vi "Main (1553).vi"() -> ()   [LabVIEW 2020]
doc: "Use this template to build a simple state machine design pattern. Each state executes code and determines which state to transition to."
uses:
  Controls/Encoding.ctl
  Controls/Database_Array.ctl
  <userlib>/_OpenG.lib/array/array.llb/Remove Duplicates from 1D Array (I32)__ogtk.vi
  <userlib>/_OpenG.lib/array/array.llb/Sort 1D Array (I32)__ogtk.vi
  <userlib>/_OpenG.lib/array/array.llb/Index 1D Array Elements (Variant)__ogtk.vi
  <userlib>/_OpenG.lib/array/array.llb/Search 1D Array (I32)__ogtk.vi
  <vilib>/Utility/error.llb/DialogType.ctl
  Libraries/Ballard_Parameter_ni/Ballard_429_Parameter_ni.lvlib
  1553/_controls/1553_State.ctl
  1553/_controls/1553_formatting.ctl
  1553/_controls/1553_Data.ctl
  1553/_controls/1553_Frames.ctl
  1553/_controls/1553_Parameters.ctl
  1553/_controls/1553_Parameters_key.ctl
  1553/_controls/1553_messages.ctl
  1553/_controls/aim1553_cluster.ctl
  Libraries/Aim_1553_Parameter_ni/AIM_1553_Parameter_ni.lvlib
panel:
  in  "formatting":T1
  in  "Configure SelfTestBus?":bool
  out "Progress":string
  in  "Stop Button":bool
  in  "Generate XMLs":bool
  in  "Database Filepath (xlsx)":path
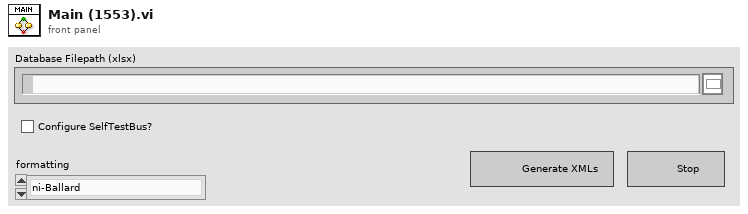
[diagram p1: front panel]
types:
  T1 = typedef "1553_formatting.ctl" = enum16{"ni-Ballard", "ni-AIM"}
  T2 = typedef "DialogType.ctl" = u16
  T3 = typedef "1553_Data.ctl" = cluster{"Cores to Process Array":i32[], "All Parameters Array":T4[], "Filtered Parameter Array":T4[], "Core Number":i32, "Database Filepath (xlsx)":path, "Selected Self Test Channels":i32[], "formatting":T1, "aim1553_cluster":T6}
  T4 = typedef "Database_Array.ctl" = cluster{"Core Number":i32, "Channel Number":i32, "Channel Name":string, "Channel Speed":i32, "Label Decimal":i32, "Label Name":string, "Min Rate (mS)":i32, "Max Rate (mS)":i32, "SDI":i32, "SSM":i32, "Create SDI":bool, "Create SSM":bool, "Create Parity":bool, "Parameter Name":string, "Start Bit":i32, "Number of Bits":i32, "Scale":string, "Offset":string, "Signed":bool, "Unit":string, "Encoding":T5, "Default Value":string}
  T5 = typedef "Encoding.ctl" = enum16{"BCD", "BNR", "Discrete"}
  T6 = typedef "aim1553_cluster.ctl" = cluster{"messages":map{string, T7}, "parameters":map{T8, T9[]}, "frames":map{string, T10}}
  T7 = typedef "1553_messages.ctl" = cluster{"messageType":string, "TA1":i32, "SA1":i32, "words":i32, "TA2":i32, "SA2":i32, "MC":i32, "direction":string}
  T8 = typedef "1553_Parameters_key.ctl" = cluster{"TA":i32, "SA":i32}
  T9 = typedef "1553_Parameters.ctl" = cluster{"name":string, "encoding":string, "signed":bool, "startBit":i32, "numberOfBits":i32, "scale":dbl, "offset":dbl, "unit":string, "defaultValue":dbl}
  T10 = typedef "1553_Frames.ctl" = cluster{"MinorFrameName":string, "MajorFrameName":string, "FramePeriodUs":i32}
  T11 = typedef "1553_State.ctl" = enum16{"Initialize", "Wait for Event", "Read Database File", "Get Core Data", "Write HW XML File", "Write Parameter XML File", "Exit"}
  T12 = enum8{"Enabled", "Disabled", "Disabled and Grayed Out"}
  T13 = enum32{"invalid app kind", "Development System", "Run Time System", "Student Edition", "Embedded LabVIEW", "Evaluation", "Custom"}
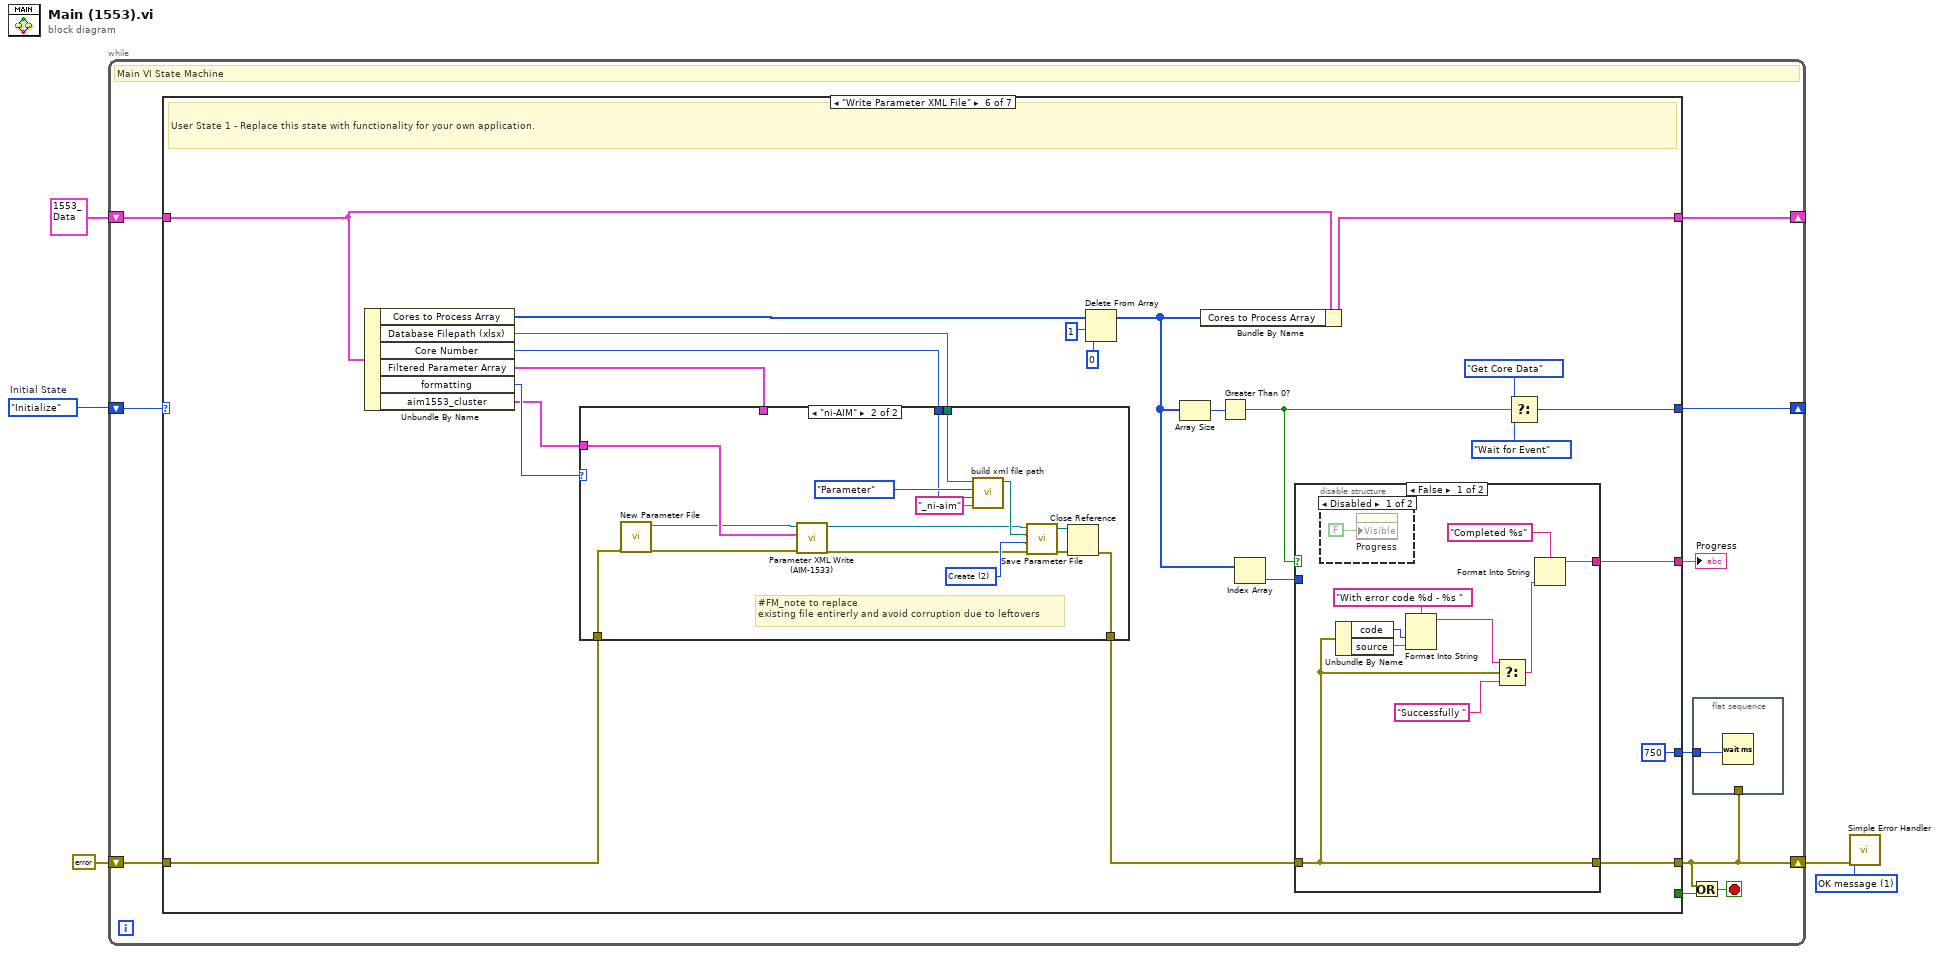
[diagram p0: block diagram]
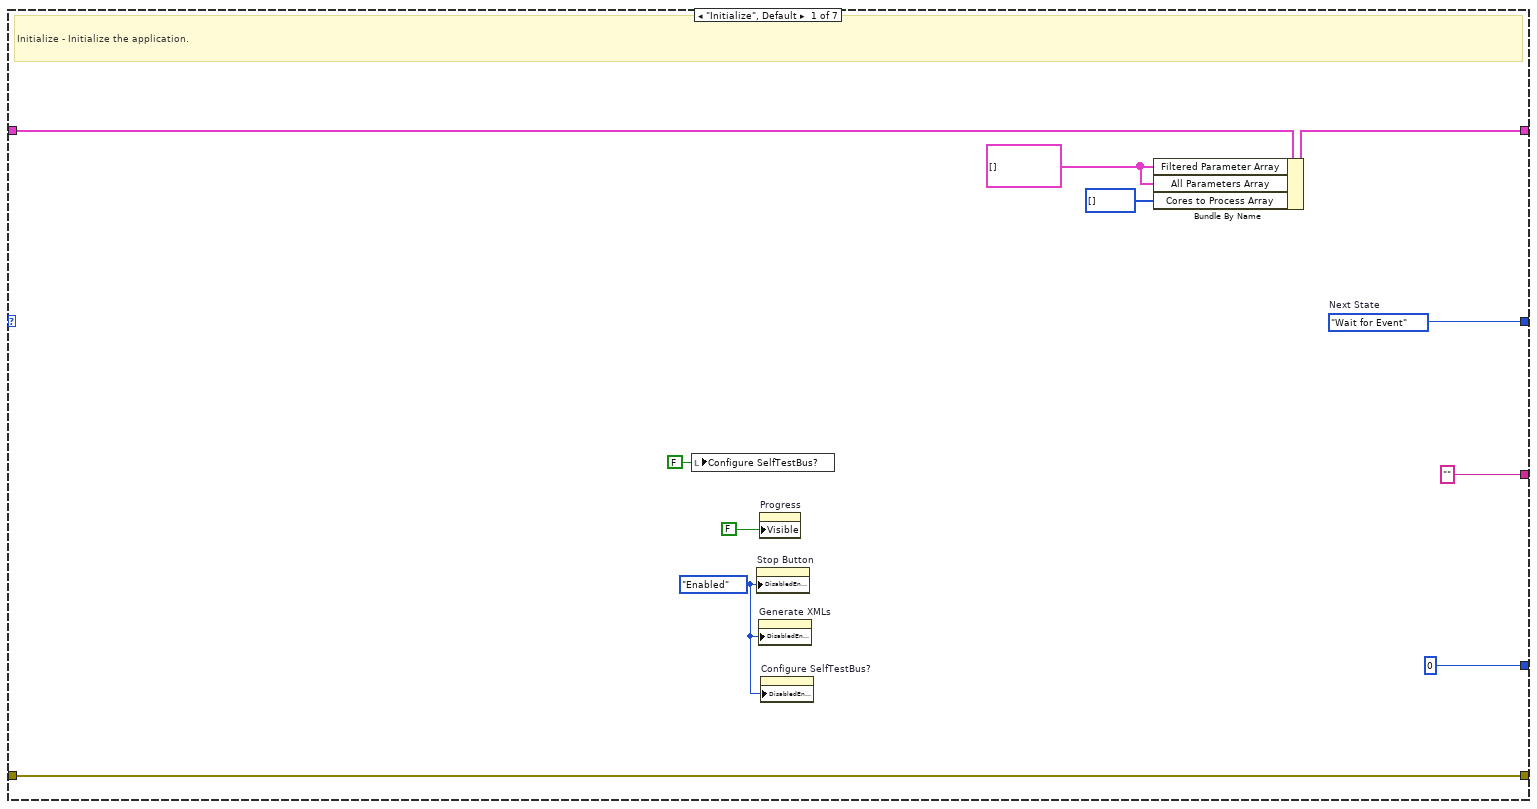
[diagram p2: hidden frame]
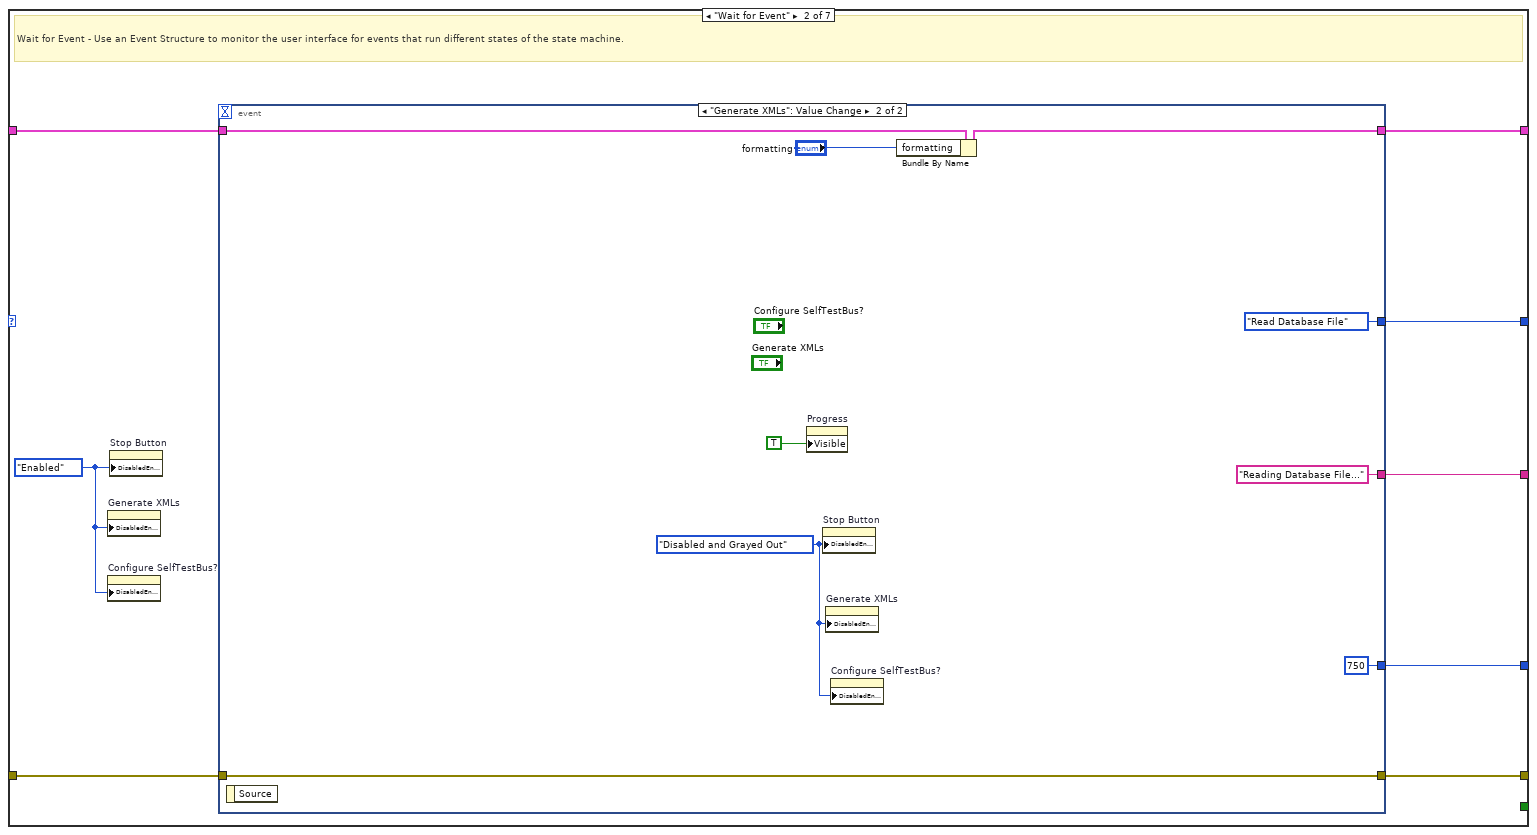
[diagram p3: hidden frame]
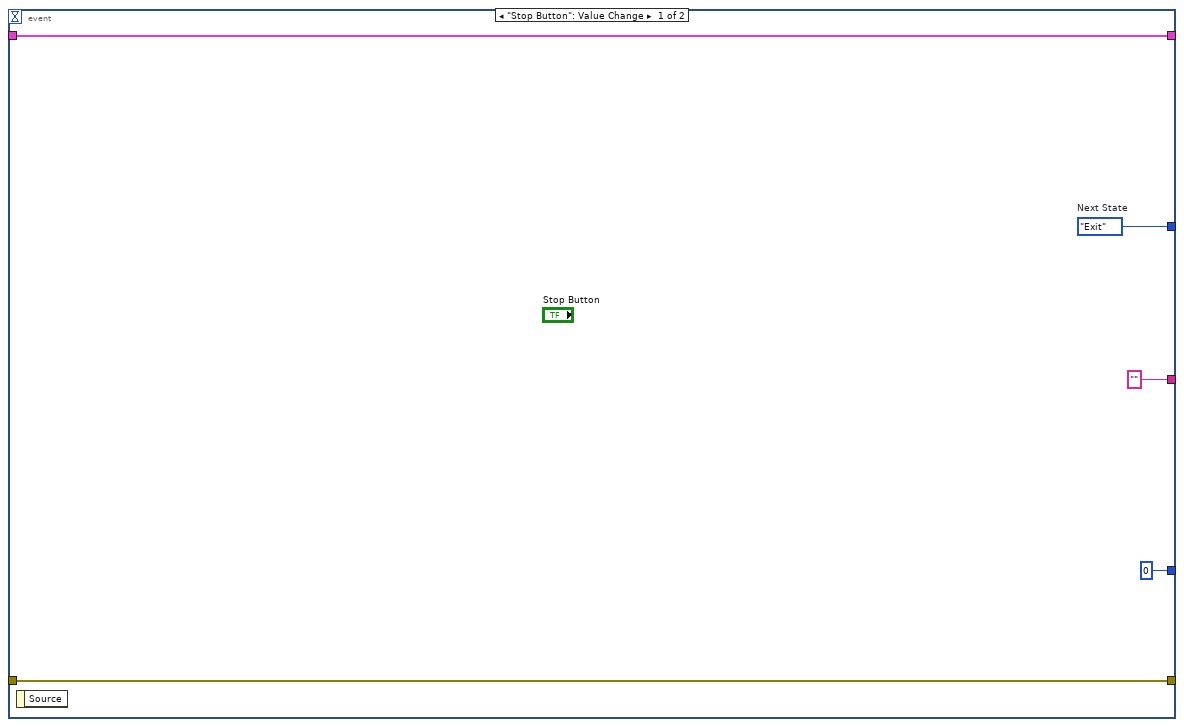
[diagram p4: hidden frame]
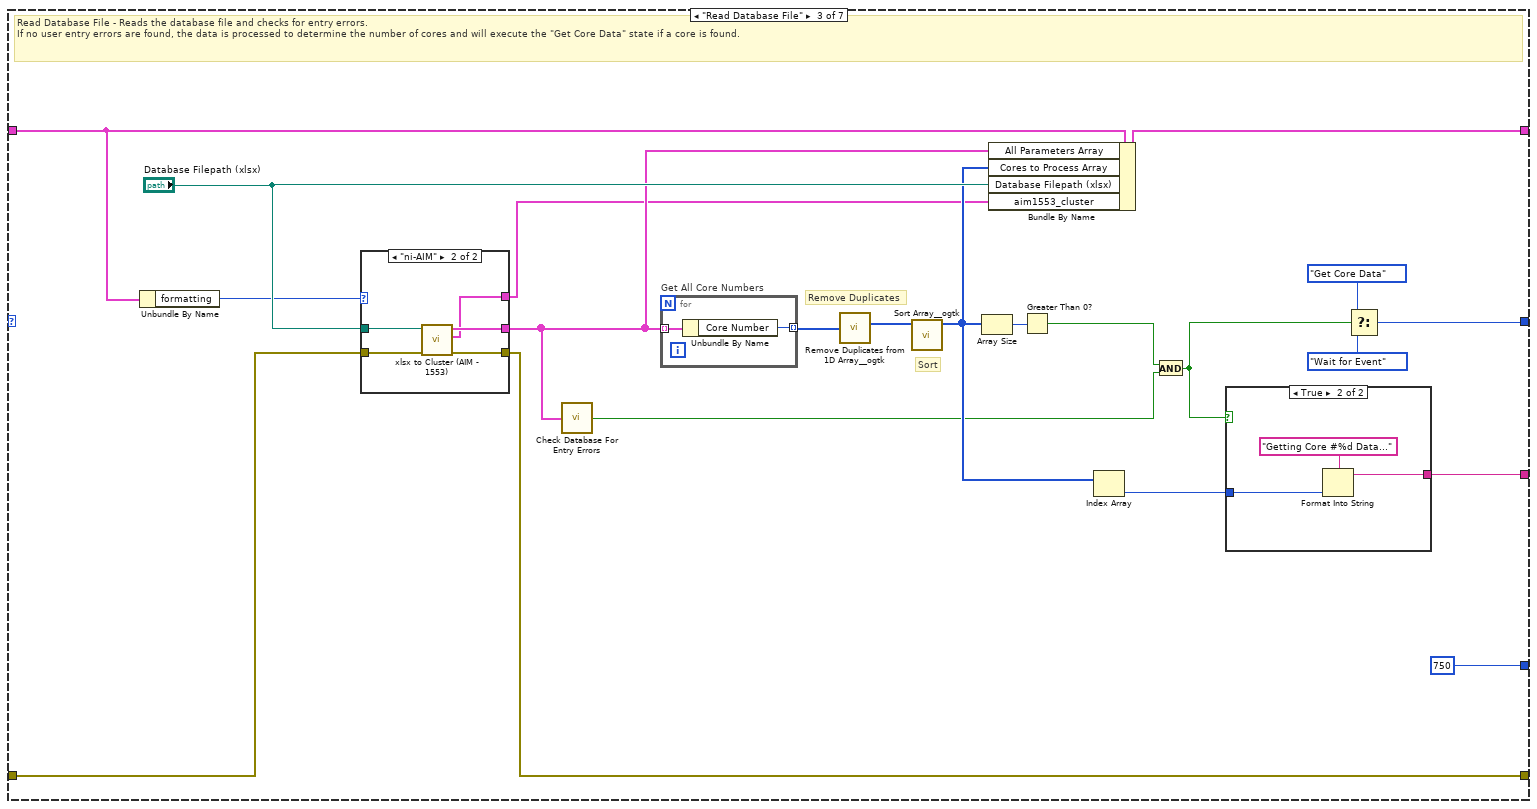
[diagram p5: hidden frame]
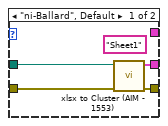
[diagram p6: hidden frame]
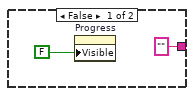
[diagram p7: hidden frame]
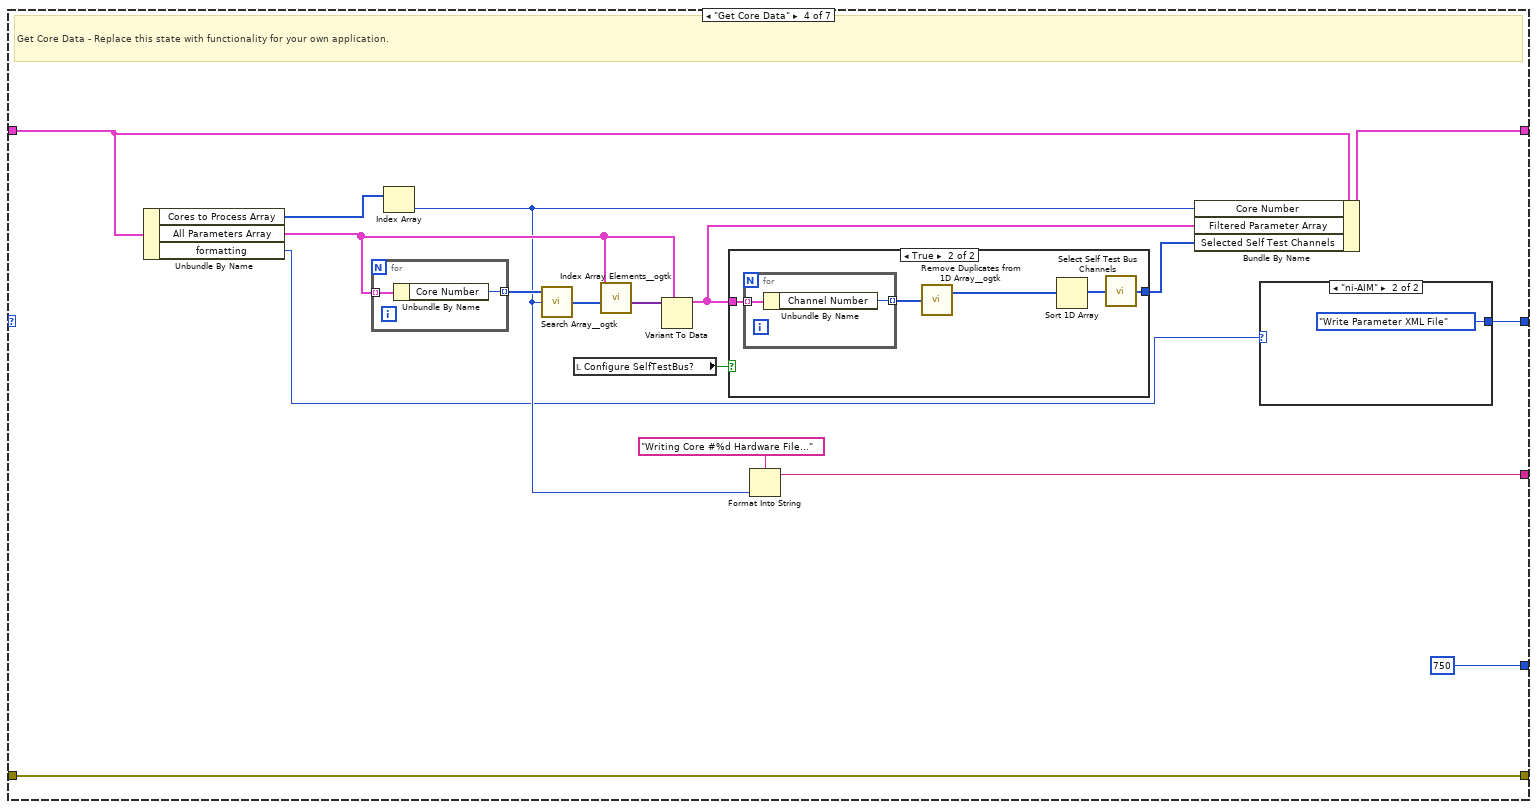
[diagram p8: hidden frame]
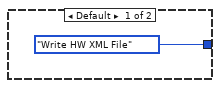
[diagram p9: hidden frame]
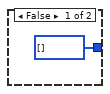
[diagram p10: hidden frame]
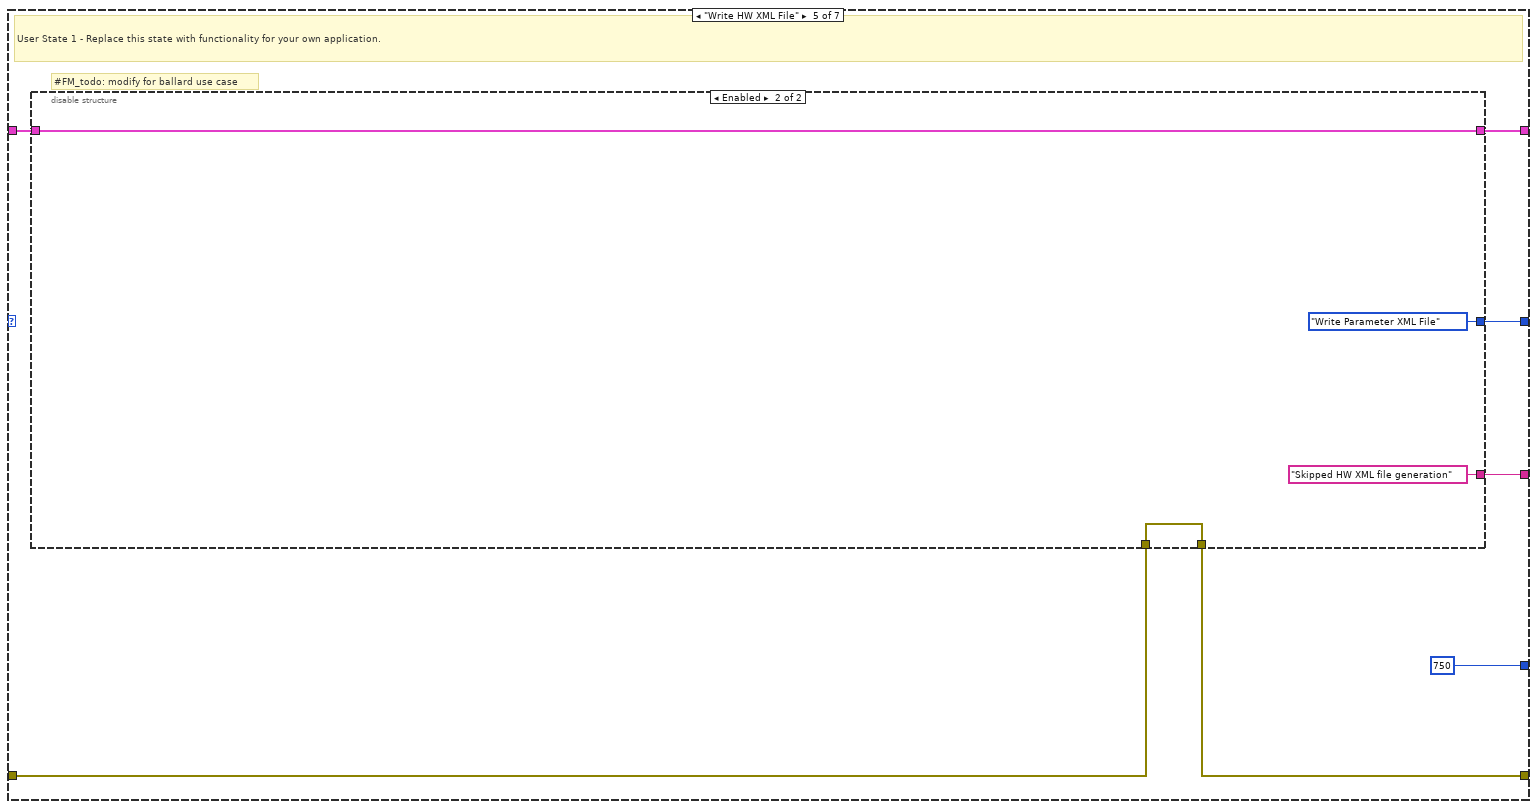
[diagram p11: hidden frame]
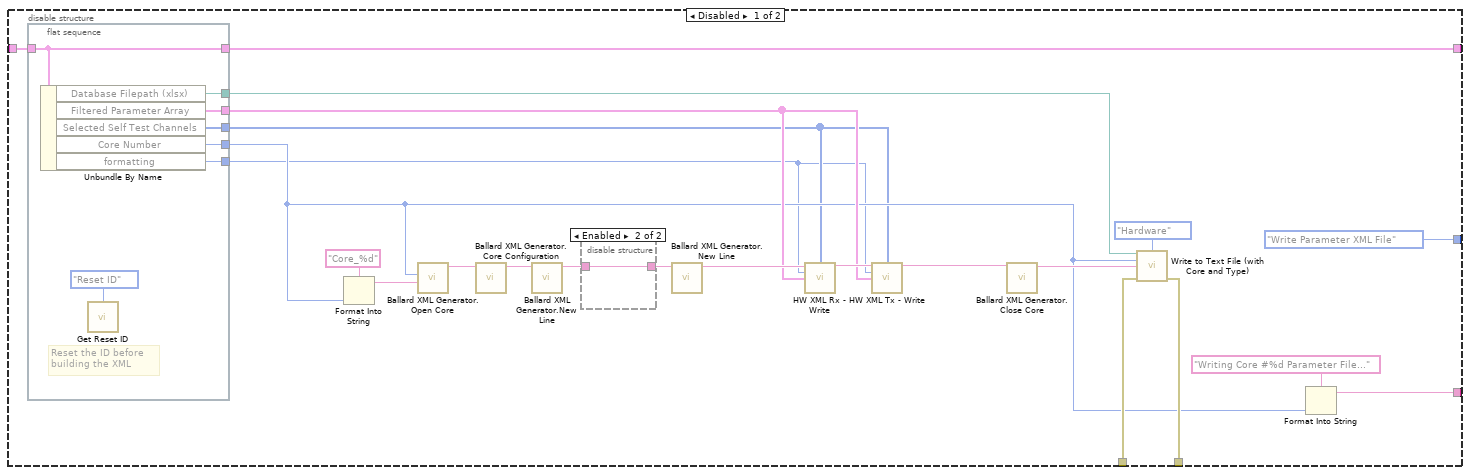
[diagram p12: hidden frame]
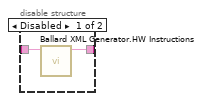
[diagram p13: hidden frame]
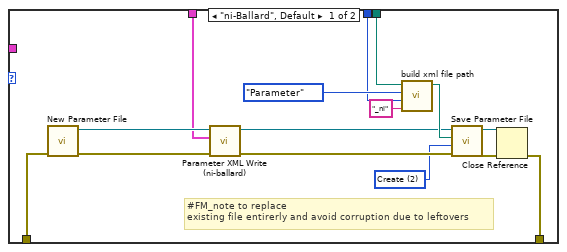
[diagram p14: hidden frame]
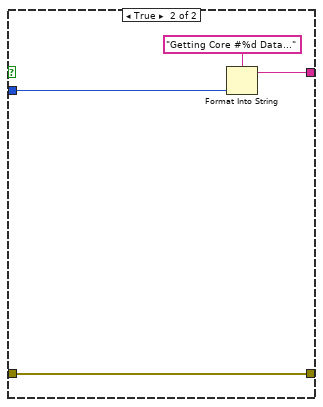
[diagram p16: hidden frame]
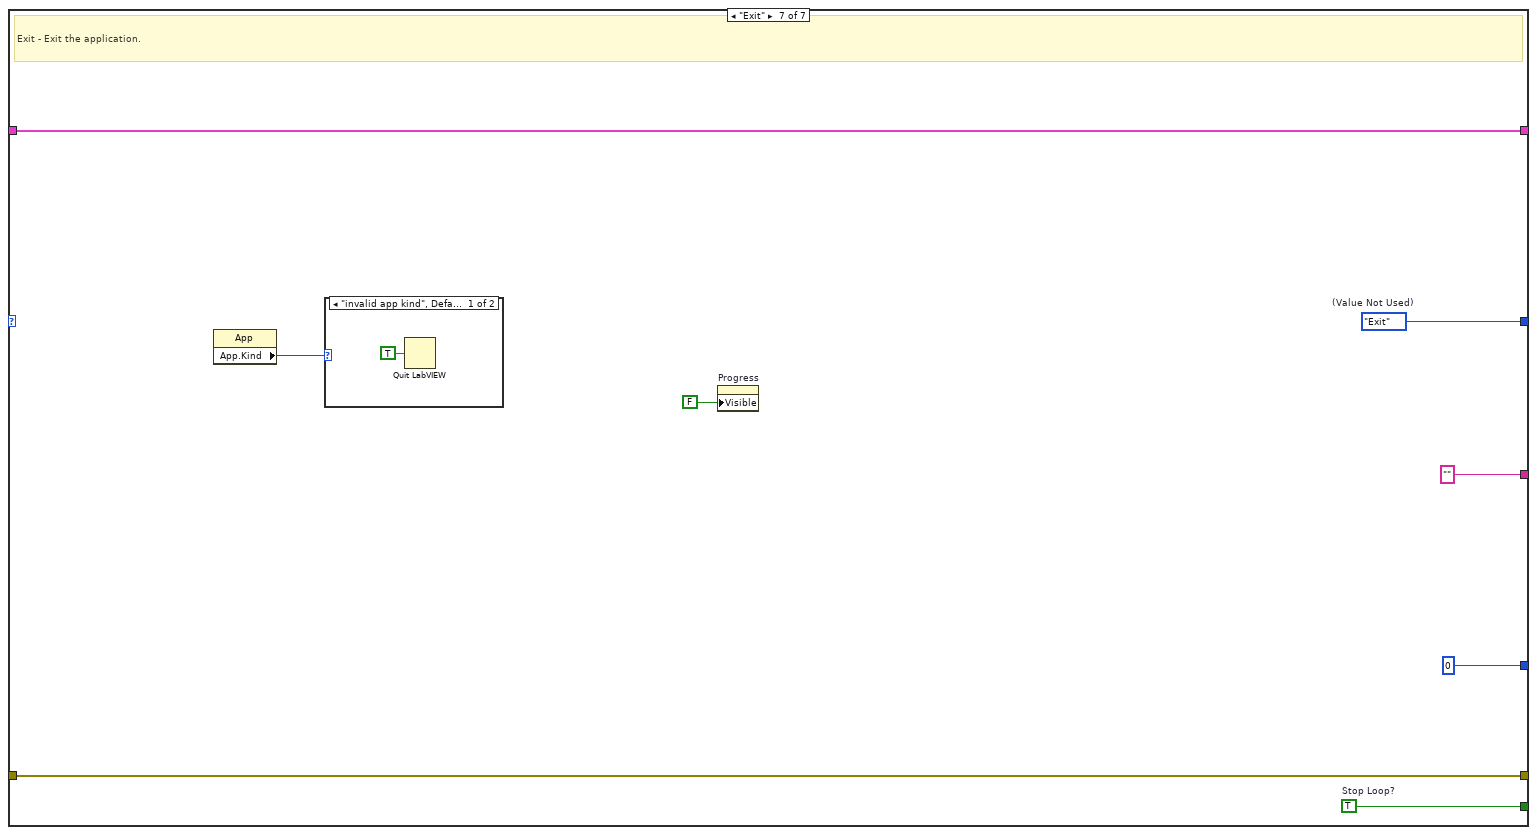
[diagram p17: hidden frame]
diagram:
  w1 = T2 1 items=["no dialog", "OK message", "continue or stop message", "OK message + warnings", "continue/stop + warnings"] ("type of dialog (OK msg:1)")
  w5 = 1553_State."Initialize"  # Initial State
  n1 = while {
    shift-right: [w14] -> _
    shift-left: w5 -> [w15]
    shift-right: [w12] -> _
    shift-left: T3 {"Cores to Process Array"=[], "All Parameters Array"=[], "Filtered Parameter Array"=[], "Core Number"=0, "Database Filepath (xlsx)"=path "C:/Users/jkreienh/Desktop/Preliminary Ballard Database Template.xlsx", "Selected Self Test Channels"=[], "formatting"=enum."ni-Ballard", "aim1553_cluster"={"messages"={}, "parameters"={}, "frames"={}}} ("Data") -> [w13]
    shift-right: [w7] -> w2
    shift-left: errorcluster {"status"=FALSE, "code"=0, "source"=""} ("error constant") -> [w11]
    stop <- w9 stop-if-true
    # "Main VI State Machine"
    n2 = case shown="\"Write Parameter XML File\"" w15 {
      tunnel: [w27 w35 w63 w97 w122 w177 w233] -> w14
      tunnel: [_ _ _ _ _ _ w231] -> w10
      tunnel: w13 -> [w25 w34 w52 w101 w119 w174 w232]
      tunnel: [w24 w33 w67 w91 w118 w173 w232] -> w12
      tunnel: w11 -> [w26 w32 w60 w96 w121 w181 w230]
      tunnel: [w26 w31 w70 w96 w120 w162 w230] -> w7
      tunnel: ["" w30 w59 w93 w117 w169 ""] -> w8
      tunnel: [u32 0 ("milliseconds to wait") w29 u32 750 ("milliseconds to wait") u32 750 ("milliseconds to wait") u32 750 ("milliseconds to wait") u32 750 ("milliseconds to wait") u32 0 ("milliseconds to wait")] -> w6
      frame "Initialize", Default {
        w18 = T12."Enabled" ("Disabled")
        w22 = T4[] [] ("Parameter Array")
        w27 = 1553_State."Wait for Event"  # Next State
        # "Initialize - Initialize the application."
        n3 = local write "Configure SelfTestBus?"(FALSE ("Configure SelfTestBus?")) -> ()
        n4 = property on="Stop Button" class="Bool"("DisabledEnum"=w18) -> ()  [unwired: 2 in, 2 out]
        n5 = property on="Generate XMLs" class="Bool"("DisabledEnum"=w18) -> ()  [unwired: 2 in, 2 out]
        n6 = property on="Progress" class="Str"("Visible"=FALSE) -> ()  [unwired: 2 in, 2 out]
        n7 = property on="Configure SelfTestBus?" class="Bool (strict)"("DisabledEnum"=w18) -> ()  [unwired: 2 in, 2 out]
        n8 = Bundle By Name(cluster=w25, "Filtered Parameter Array"=w22, "All Parameters Array"=w22, "Cores to Process Array"=i32[] [] ("Core Array")) -> (w24:T3)
      }
      frame "Wait for Event" {
        w28 = T12."Enabled" ("Disabled")
        # "Wait for Event - Use an Event Structure to monitor the user interface for events that run different states of the state machine."
        n9 = property on="Generate XMLs" class="Bool"("DisabledEnum"=w28) -> ()  [unwired: 2 in, 2 out]
        n10 = property on="Configure SelfTestBus?" class="Bool (strict)"("DisabledEnum"=w28) -> ()  [unwired: 2 in, 2 out]
        n11 = property on="Stop Button" class="Bool"("DisabledEnum"=w28) -> ()  [unwired: 2 in, 2 out]
        n12 = event shown="[1] \"Generate XMLs\": Value Change" {
          selector: _ -> [_ _]
          dyn-events: _ -> [_ _]
          timeout: _ -> [_ _]
          tunnel: [w40 1553_State."Read Database File" ("Next State")] -> w35
          tunnel: w34 -> [w39 w49]
          tunnel: [w39 w42] -> w33
          tunnel: w32 -> [w38 w48]
          tunnel: [w38 w48] -> w31
          tunnel: ["" "Reading Database File..."] -> w30
          tunnel: [u32 0 ("milliseconds to wait") u32 750 ("milliseconds to wait")] -> w29
          event "Stop Button": Value Change {
            w40 = 1553_State."Exit"  # Next State
            n13 = event-data() -> ()  [unwired: 1 in, 1 out]
          }
          event "Generate XMLs": Value Change {
            w43 = T12."Disabled and Grayed Out" ("Disabled")
            n14 = event-data() -> ()  [unwired: 1 in, 1 out]
            n15 = property on="Progress" class="Str"("Visible"=TRUE) -> ()  [unwired: 2 in, 2 out]
            n16 = property on="Stop Button" class="Bool"("DisabledEnum"=w43) -> ()  [unwired: 2 in, 2 out]
            n17 = property on="Generate XMLs" class="Bool"("DisabledEnum"=w43) -> ()  [unwired: 2 in, 2 out]
            n18 = property on="Configure SelfTestBus?" class="Bool (strict)"("DisabledEnum"=w43) -> ()  [unwired: 2 in, 2 out]
            n19 = Bundle By Name(cluster=w49, "formatting"="formatting") -> (w42:T3)
          }
        }
      }
      frame "Read Database File" {
        # "Sort"
        # "Remove Duplicates"
        # "Read Database File - Reads the database file and checks for entry errors. \nIf no user entry errors are found, the data is processed to determine the number of cores and will execute the \"Get Core Data\" state if a core is found."
        n20 = Unbundle By Name(w52) -> ("formatting"=w51:T1)
        n21 = case shown="\"ni-AIM\"" w51 {
          tunnel: [w74 w77] -> w70
          tunnel: "Database Filepath (xlsx)" -> [w73 w79]
          tunnel: [w72 w76] -> w61
          tunnel: w60 -> [w71 w78]
          tunnel: [_ w75] -> w50
          frame "ni-Ballard", Default {
            (unwired) "Sheet1" ("Excel._SheetName")
            n22 = call "xlsx to Cluster (AIM - 1553).vi"("Error (in)"=w71, "file path (dialog if empty)"=w73) -> ("Error (out)"=w74:errorcluster, "Parameter Array"=w72:T4[])  [unwired: 7 in, 1 out]
          }
          frame "ni-AIM" {
            n23 = call "xlsx to Cluster (AIM - 1553).vi"("Error (in)"=w78, "file path (dialog if empty)"=w79) -> ("Error (out)"=w77:errorcluster, "aim1553_cluster"=w75:T6, "Parameter Array"=w76:T4[])  [unwired: 7 in]
          }
        }
        n24 = call "Check Database For Entry Errors.vi"("All Parameters Array"=w61) -> ("Database OK?"=w54:bool)  [unwired: 14 in]
        n25 = for "Get All Core Numbers" {
          tunnel: w61 -> [w86] mode=indexing
          tunnel: [w85] -> w69 mode=indexing
          n26 = Unbundle By Name(w86) -> ("Core Number"=w85:i32)
        }
        n27 = call-poly <userlib>:"Remove Duplicates from 1D Array__ogtk.vi"("Input Array"=w69) -> ("Output Array"=w68:i32[])  [unwired: 1 out]
        n28 = call-poly <userlib>:"Sort Array__ogtk.vi"("Array in"=w68) -> ("Sorted Array out"=w58:i32[])  [unwired: 9 in, 1 out]
        n29 = Array Size(array=w58) -> (size(s)=w66:i32)
        n30 = Bundle By Name(cluster=w52, "All Parameters Array"=w61, "Cores to Process Array"=w58, "Database Filepath (xlsx)"="Database Filepath (xlsx)", "aim1553_cluster"=w50) -> (w67:T3)
        n31 = Greater Than 0?(x=w66) -> (x > 0?=w55:bool)
        n32 = Index Array(array=w58) -> (element=w57:i32)  [unwired: 1 in]
        n33 = And(x=w55, y=w54) -> (x .and. y?=w53:bool)
        n34 = case shown="True" w53 {
          tunnel: ["" ("f") w83] -> w59
          tunnel: w57 -> [_ w84]
          frame False {
            n35 = property on="Progress" class="Str"("Visible"=FALSE) -> ()  [unwired: 2 in, 2 out]
          }
          frame True {
            n36 = Format Into String(format string="Getting Core #%d Data..." ("String"), w84) -> (resulting string=w83:string)  [unwired: 2 in, 1 out]
          }
        }
        n37 = Select(t=1553_State."Get Core Data", s=w53, f=1553_State."Wait for Event") -> (s? t:f=w63:T11)
      }
      frame "Get Core Data" {
        # "Get Core Data - Replace this state with functionality for your own application."
        n38 = Unbundle By Name(w101) -> ("Cores to Process Array"=w98:i32[], "All Parameters Array"=w100:T4[], "formatting"=w87:T1)
        n39 = for {
          tunnel: w100 -> [w115] mode=indexing
          tunnel: [w114] -> w103 mode=indexing
          n40 = Unbundle By Name(w115) -> ("Core Number"=w114:i32)
        }
        n41 = Index Array(array=w98) -> (element=w94:i32)  [unwired: 1 in]
        n42 = call-poly <userlib>:"Search Array__ogtk.vi"("Array"=w103, "Element Data"=w94) -> ("Indices of Elements"=w102:i32[])  [unwired: 7 in]
        n43 = local read "Configure SelfTestBus?"() -> (w88:bool)
        n44 = call-poly <userlib>:"Index Array Elements__ogtk.vi"("indices"=w102, "array"=w100) -> ("elements"=w99:variant[])  [unwired: 9 in]
        n45 = Variant To Data(type=w100, Variant=w99) -> (data=w90:T4[])  [unwired: 1 in, 1 out]
        n46 = case shown="True" w88 {
          tunnel: w90 -> [_ w110]
          tunnel: [i32[] [] ("Selected Channels") w107] -> w89
          frame False {
          }
          frame True {
            n47 = for {
              tunnel: [w113] -> w109 mode=indexing
              tunnel: w110 -> [w112] mode=indexing
              n48 = Unbundle By Name(w112) -> ("Channel Number"=w113:i32)
            }
            n49 = call-poly <userlib>:"Remove Duplicates from 1D Array__ogtk.vi"("Input Array"=w109) -> ("Output Array"=w111:i32[])  [unwired: 1 out]
            n50 = Sort 1D Array(array=w111) -> (sorted array=w108:i32[])
            n51 = call "Select Self Test Bus Channels.vi"("Channels"=w108) -> ("Selected Channels"=w107:i32[])  [unwired: 14 in]
          }
        }
        n52 = Format Into String(format string="Writing Core #%d Hardware File..." ("String"), w94) -> (resulting string=w93:string)  [unwired: 2 in, 1 out]
        n53 = Bundle By Name(cluster=w101, "Core Number"=w94, "Filtered Parameter Array"=w90, "Selected Self Test Channels"=w89) -> (w91:T3)
        n54 = case shown="\"ni-AIM\"" w87 {
          tunnel: [1553_State."Write HW XML File" 1553_State."Write Parameter XML File"] -> w97
          frame Default {
          }
          frame "ni-AIM" {
          }
        }
      }
      frame "Write HW XML File" {
        # "#FM_todo: modify for ballard use case"
        # "User State 1 - Replace this state with functionality for your own application."
        n55 = disable-structure shown="Enabled" {
          disable-tunnel: [1553_State."Write Parameter XML File" ("Next State") 1553_State."Write Parameter XML File" ("Next State")] -> w122
          disable-tunnel: w121 -> [w133 w157]
          disable-tunnel: [w132 w157] -> w120
          disable-tunnel: w119 -> [w130 w158]
          disable-tunnel: [w129 w158] -> w118
          disable-tunnel: [w126 "Skipped HW XML file generation"] -> w117
          frame Disabled {
            n56 = flat-sequence {
              tunnel: [w152] -> w135
              tunnel: w130 -> [w150]
              tunnel: [w150] -> w129
              tunnel: [w149] -> w128
              tunnel: [w148] -> w125
              tunnel: [w147] -> w124
              tunnel: [w146] -> w123
              frame #0 {
                # "Reset the ID before building the XML"
                n57 = Unbundle By Name(w150) -> ("Database Filepath (xlsx)"=w149:path, "Filtered Parameter Array"=w152:T4[], "Selected Self Test Channels"=w147:i32[], "Core Number"=w148:i32, "formatting"=w146:T1)
                n58 = call "Get Reset ID.vi"("Function"=enum16{"Get ID", "Reset ID"}."Reset ID") -> ()  [unwired: 14 in, 1 out]
              }
            }
            n59 = Format Into String(format string="Core_%d", w125) -> (resulting string=w136:string)  [unwired: 2 in, 1 out]
            n60 = call "Ballard XML Generator.Open Core.vi"("name"=w136, "id"=w125) -> ("string out"=w138:string)  [unwired: 9 in]
            n61 = call "Ballard XML Generator.Core Configuration.vi"("string in"=w138) -> ("string out"=w139:string)  [unwired: 10 in]
            n62 = call "Ballard XML Generator.New Line.vi"("string in"=w139) -> ("string out"=w140:string)  [unwired: 10 in]
            n63 = disable-structure shown="Enabled" {
              disable-tunnel: w140 -> [w154 w155]
              disable-tunnel: [w153 w155] -> w141
              frame Disabled {
                n64 = call "Ballard XML Generator.HW Instructions.vi"("string in"=w154) -> ("string out"=w153:string)  [unwired: 10 in]
              }
              frame Enabled {
              }
            }
            n65 = call "Ballard XML Generator.New Line.vi"("string in"=w141) -> ("string out"=w142:string)  [unwired: 10 in]
            n66 = call "HW XML Rx - Write.vi"("String (in)"=w142, "Selected Channels"=w124, "formatting (NIVeriStandAdd-Ons)"=w123, "Parameter Array"=w135) -> ("String (out)"=w143:string)  [unwired: 11 in]
            n67 = call "HW XML Tx - Write.vi"("String (in)"=w143, "Selected Channels"=w124, "formatting (NIVeriStandAdd-Ons)"=w123, "Parameter Array"=w135) -> ("String (out)"=w144:string)  [unwired: 11 in]
            n68 = call "Ballard XML Generator.Close Core.vi"("string in"=w144) -> ("string out"=w131:string)  [unwired: 10 in]
            n69 = call "Write to Text File (with Core and Type).vi"("Database Filepath (xlsx)"=w128, "Filetype"=enum16{"Hardware", "Parameter"}."Hardware", "Core"=w125, "Text"=w131, "Error (in)"=w133) -> ("Error (out)"=w132:errorcluster)  [unwired: 10 in]
            n70 = Format Into String(format string="Writing Core #%d Parameter File..." ("String"), w125) -> (resulting string=w126:string)  [unwired: 2 in, 1 out]
          }
          frame Enabled {
          }
        }
      }
      frame "Write Parameter XML File" {
        # "User State 1 - Replace this state with functionality for your own application."
        n71 = Unbundle By Name(w174) -> ("Cores to Process Array"=w175:i32[], "Database Filepath (xlsx)"=w171:path, "Core Number"=w168:i32, "Filtered Parameter Array"=w172:T4[], "formatting"=w161:T1, "aim1553_cluster"=w160:T6)
        n72 = case shown="\"ni-AIM\"" w161 {
          tunnel: w181 -> [w196 w205]
          tunnel: [w195 w211] -> w163
          tunnel: w172 -> [w186 _]
          tunnel: w171 -> [w191 w209]
          tunnel: w168 -> [w190 w208]
          tunnel: w160 -> [_ w206]
          frame "ni-Ballard", Default {
            w182 = 2 items=["CreateNew"=1, "Create"=2, "Open"=3, "OpenOrCreate"=4, "Truncate"=5, "Append"=6] ("mode (Create)")
            # "#FM_note to replace \nexisting file entirerly and avoid corruption due to leftovers"
            n73 = call "New Parameter File.vi"("error in"=w196) -> ("error out"=w187:errorcluster, "new parameter file"=w188:refnum<k24>)  [unwired: 9 in]
            n74 = call "Parameter XML Write (ni-ballard).vi"("error in"=w187, "Parameter Array"=w186, "parameter file in"=w188) -> ("error out"=w184:errorcluster, "parameter file out"=w185:refnum<k24>)  [unwired: 7 in]
            n75 = call "build xml file path.vi"("additional string(\"\")"="_ni" ("additional string(\"\")"), "Core"=w190, "Filetype"=enum16{"Hardware", "Parameter"}."Parameter", "Database Filepath in"=w191) -> ("xml path out"=w189:path)  [unwired: 7 in]
            n76 = call "Save Parameter File.vi"("error in"=w184, "mode (Create)"=w182, "XML path"=w189, "parameter file in"=w185) -> ("error out"=w194:errorcluster, "parameter file out"=w193:refnum<k24>)  [unwired: 5 in, 1 out]
            n77 = Close Reference(reference=w193, error in (no error)=w194) -> (error out=w195:errorcluster)
          }
          frame "ni-AIM" {
            w202 = 2 items=["CreateNew"=1, "Create"=2, "Open"=3, "OpenOrCreate"=4, "Truncate"=5, "Append"=6] ("mode (Create)")
            # "#FM_note to replace \nexisting file entirerly and avoid corruption due to leftovers"
            n78 = call "New Parameter File.vi"("error in"=w205) -> ("error out"=w198:errorcluster, "new parameter file"=w197:refnum<k24>)  [unwired: 9 in]
            n79 = call "Parameter XML Write (AIM-1533).vi"("error in"=w198, "aim1553_cluster"=w206, "parameter file in"=w197) -> ("error out"=w200:errorcluster, "parameter file out"=w199:refnum<k24>)  [unwired: 7 in]
            n80 = call "build xml file path.vi"("additional string(\"\")"="_ni-aim" ("additional string(\"\")"), "Core"=w208, "Filetype"=enum16{"Hardware", "Parameter"}."Parameter", "Database Filepath in"=w209) -> ("xml path out"=w201:path)  [unwired: 7 in]
            n81 = call "Save Parameter File.vi"("error in"=w200, "mode (Create)"=w202, "XML path"=w201, "parameter file in"=w199) -> ("error out"=w204:errorcluster, "parameter file out"=w203:refnum<k24>)  [unwired: 5 in, 1 out]
            n82 = Close Reference(reference=w203, error in (no error)=w204) -> (error out=w211:errorcluster)
          }
        }
        n83 = Delete From Array(array=w175, length=1, index=0) -> (array with subset deleted=w166:i32[])  [unwired: 1 out]
        n84 = Array Size(array=w166) -> (size(s)=w180:i32)
        n85 = Bundle By Name(cluster=w174, "Cores to Process Array"=w166) -> (w173:T3)
        n86 = Greater Than 0?(x=w180) -> (x > 0?=w167:bool)
        n87 = Index Array(array=w166) -> (element=w165:i32)  [unwired: 1 in]
        n88 = case shown="False" w167 {
          tunnel: [w219 w224] -> w169
          tunnel: w165 -> [_ w223]
          tunnel: w163 -> [w212 w222]
          tunnel: [w212 w222] -> w162
          frame False {
            n89 = disable-structure shown="Disabled" {
              frame Disabled {
                n90 = property on="Progress" class="Str"("Visible"=FALSE) -> ()  [unwired: 2 in, 2 out]
              }
              frame Enabled {
              }
            }
            n91 = Unbundle By Name(w212) -> ("code"=w217:i32, "source"=w216:string)
            n92 = Format Into String(format string="With error code %d - %s ", w217, w216) -> (resulting string=w214:string)  [unwired: 2 in, 1 out]
            n93 = Select(t=w214, s=w212, f="Successfully ") -> (s? t:f=w215:string)
            n94 = Format Into String(format string="Completed %s", w215) -> (resulting string=w219:string)  [unwired: 2 in, 1 out]
          }
          frame True {
            n95 = Format Into String(format string="Getting Core #%d Data..." ("String"), w223) -> (resulting string=w224:string)  [unwired: 2 in, 1 out]
          }
        }
        n96 = Select(t=1553_State."Get Core Data" ("Next State"), s=w167, f=1553_State."Wait for Event" ("Next State")) -> (s? t:f=w177:T11)
      }
      frame "Exit" {
        w231 = TRUE  # Stop Loop?
        w233 = 1553_State."Exit"  # (Value Not Used)
        # "Exit - Exit the application."
        n97 = property class="App"() -> ("App.Kind"=w226:T13)  [unwired: 2 in, 2 out]
        n98 = case shown="\"invalid app kind\", Default" w226 {
          frame "invalid app kind", Default {
            n99 = Quit LabVIEW(quit? (T)=TRUE) -> ()
          }
          frame "Development System" {
          }
        }
        n100 = property on="Progress" class="Str"("Visible"=FALSE) -> ()  [unwired: 2 in, 2 out]
      }
    }
    "Progress" <- w8
    n101 = Or(x=w7, y=w10) -> (x .or. y?=w9:bool)
    n102 = flat-sequence {
      tunnel: w7 -> [_]
      tunnel: w6 -> [w16]
      frame #0 {
        n103 = Wait (ms)(milliseconds to wait=w16) -> ()  [unwired: 1 out]
      }
    }
  }
  n104 = call <vilib>:"Simple Error Handler.vi"("type of dialog (OK msg:1)"=w1, "error in (no error)"=w2) -> ()  [unwired: 3 in, 5 out]
